vi "Velocity Sensor Data.vi"(8 "Error":errorcluster, 11 "Motor Follow":T3) -> (0 "Error Out":errorcluster, 1 "Voltage Data":T1, 2 "Velocity Data (RPM) Out":T2, 3 "PhoenixMotorControlDevRef Out":T3)   [LabVIEW 2023, in "ChainLift_ACT.lvlib"]
uses:
  ChainLift_ACT.lvlib
  <vilib>/Rock Robotics/SystemInterfaces/DIO/FPGA_DIOPWMChannel.ctl
  <vilib>/Rock Robotics/WPI/PWM/WPI_PWMDeadband.ctl
  <vilib>/Rock Robotics/WPI/MotorControl/WPI_MotorControlType.ctl
  <vilib>/Rock Robotics/SystemInterfaces/DIO/FPGA_DIOChannel.ctl
  <vilib>/Rock Robotics/WPI/MotorControl/WPI_MotorControlDeviceRef.ctl
  Cluster_Velocity Values.ctl
  Cluster_Voltage Values.ctl
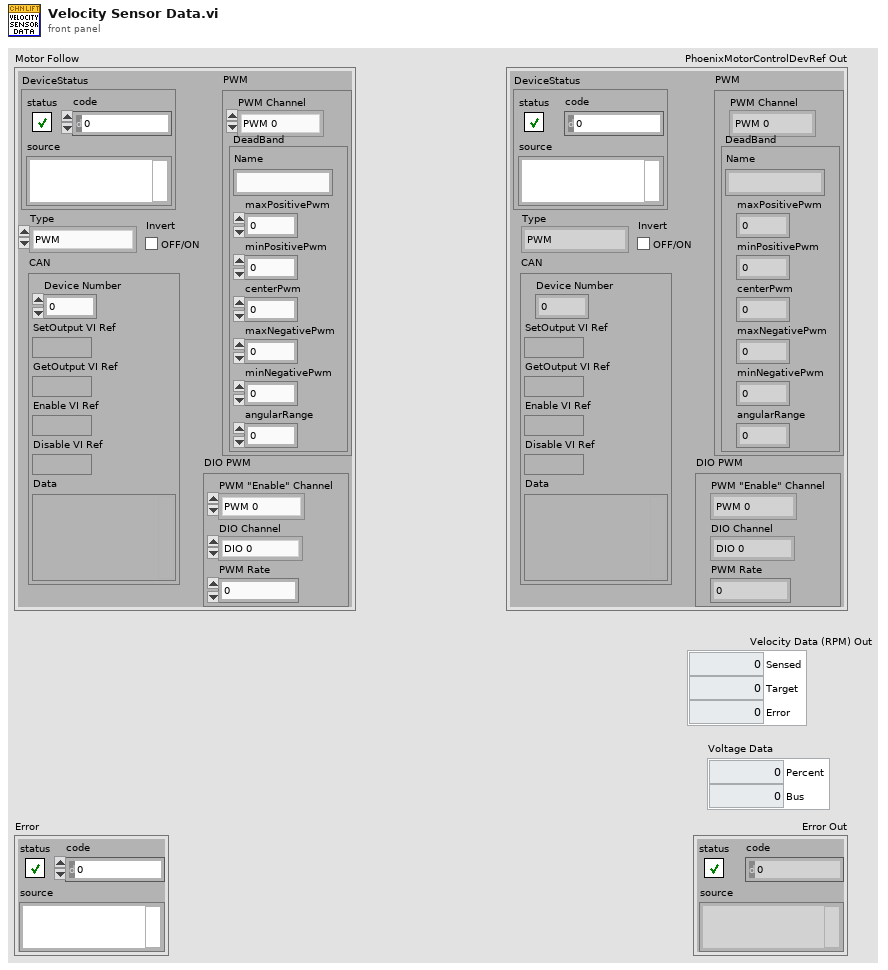
[diagram p1: front panel]
types:
  T1 = typedef "ChainLift_ACT.lvlib/Cluster_Voltage Values.ctl" = cluster{"Percent":dbl, "Bus":dbl}
  T2 = typedef "ChainLift_ACT.lvlib/Cluster_Velocity Values.ctl" = cluster{"Sensed":dbl, "Target":dbl, "Error":dbl}
  T3 = typedef "WPI_MotorControlDeviceRef.ctl" = cluster{"DeviceStatus":errorcluster, "Type":T4, "PWM":cluster{"PWM Channel":T5, "DeadBand":T6}, "CAN":cluster{"Device Number":u8, "SetOutput VI Ref":variant, "GetOutput VI Ref":variant, "Enable VI Ref":variant, "Disable VI Ref":variant, "Data":variant}, "Invert":bool, "DIO PWM":cluster{"PWM \"Enable\" Channel":T5, "DIOChannel":T7, "PWM Rate":dbl}}
  T4 = typedef "WPI_MotorControlType.ctl" = enum16{"PWM", "CAN", "DIO PWM"}
  T5 = typedef "FPGA_DIOPWMChannel.ctl" = enum8{"PWM 0", "PWM 1", "PWM 2", "PWM 3", "PWM 4", "PWM 5", "PWM 6", "PWM 7", "PWM 8", "PWM 9", "PWM MXP 0", "PWM MXP 1", "PWM MXP 2", "PWM MXP 3", "PWM MXP 4", "PWM MXP 5", "PWM MXP 6", "PWM MXP 7", "PWM MXP 8", "PWM MXP 9", "Invalid"}
  T6 = typedef "WPI_PWMDeadband.ctl" = cluster{"Name":string, "maxPositivePwm":i32, "minPositivePwm":i32, "centerPwm":i32, "maxNegativePwm":i32, "minNegativePwm":i32, "angularRange":u16}
  T7 = typedef "FPGA_DIOChannel.ctl" = enum8{"DIO 0", "DIO 1", "DIO 2", "DIO 3", "DIO 4", "DIO 5", "DIO 6", "DIO 7", "DIO 8", "DIO 9", "DIO MXP 0", "DIO MXP 1", "DIO MXP 2", "DIO MXP 3", "DIO MXP 4", "DIO MXP 5", "DIO MXP 6", "DIO MXP 7", "DIO MXP 8", "DIO MXP 9", "DIO MXP 10", "DIO MXP 11", "DIO MXP 12", "DIO MXP 13", "DIO MXP 14", "DIO MXP 15", "SPI Port CS1", "SPI Port CS2", "SPI Port CS3", "SPI Port MISO", "SPI Port MOSI", "Invalid"}
  T8 = typedef "Cluster_Speed Sensor Values.ctl" = cluster{"Velocity":T9, "Voltage":T10}
  T9 = typedef "Shooter_ACT.lvlib/Cluster_Velocity Values.ctl" = cluster{"Sensed":dbl, "Target":dbl, "Error":dbl}
  T10 = typedef "Shooter_ACT.lvlib/Cluster_Voltage Values.ctl" = cluster{"Percent":dbl, "Bus":dbl}
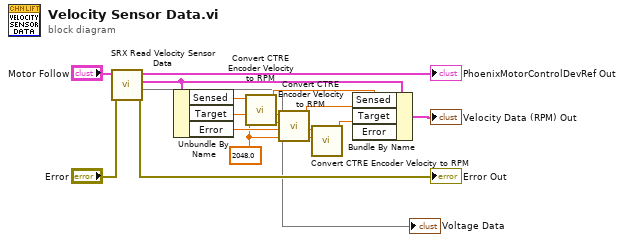
[diagram p0: block diagram]
diagram:
  w2 = 2048.0 ("Units/ Rev")
  n1 = call "SRX Read Velocity Sensor Data.vi"("Error"="Error", "SRX Ref"="Motor Follow") -> ("Error Out"=→"Error Out":errorcluster, 1:→"Voltage Data", "Sensor Status Out"=w13:T8, "SRX Ref Out"=→"PhoenixMotorControlDevRef Out":T3)  [unwired: 6 in]
  n2 = Unbundle By Name(w13) -> ("Sensed"=w14:dbl, "Target"=w6:dbl, "Error"=w5:dbl)
  n3 = call "Convert CTRE Encoder Velocity to RPM.vi"("Units/ Rev"=w2, "CTRE Vel (units/.1S)"=w14) -> ("RPM Out"=w7:dbl)  [unwired: 9 in]
  n4 = call "Convert CTRE Encoder Velocity to RPM.vi"("Units/ Rev"=w2, "CTRE Vel (units/.1S)"=w6) -> ("RPM Out"=w4:dbl)  [unwired: 9 in]
  n5 = call "Convert CTRE Encoder Velocity to RPM.vi"("Units/ Rev"=w2, "CTRE Vel (units/.1S)"=w5) -> ("RPM Out"=w3:dbl)  [unwired: 9 in]
  n6 = Bundle By Name(cluster=w13, "Sensed"=w7, "Target"=w4, "Error"=w3) -> (→"Velocity Data (RPM) Out":T8)
